vi "Keithley24xx_qMeasVil.vi"(5 "Vih, V":dbl, 6 "Vil, V":dbl, 7 "Voh, V":dbl, 8 "outVISA In":refnum<visa-resource-name>, 9 "outErr In":errorcluster, 10 "inVISA In":refnum<visa-resource-name>, 11 "inErr In":errorcluster) -> (0 "outVISA Out":refnum<visa-resource-name>, 1 "outErr Out":errorcluster, 2 "inVISA Out":refnum<visa-resource-name>, 3 "inErr Out":errorcluster, 4 "Vil meas, В":dbl format="%#.3g")   [LabVIEW 2014]
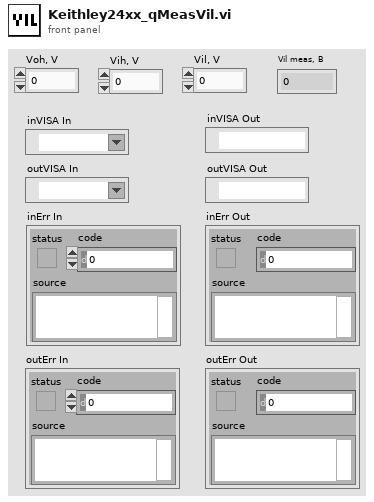
[diagram p1: front panel]
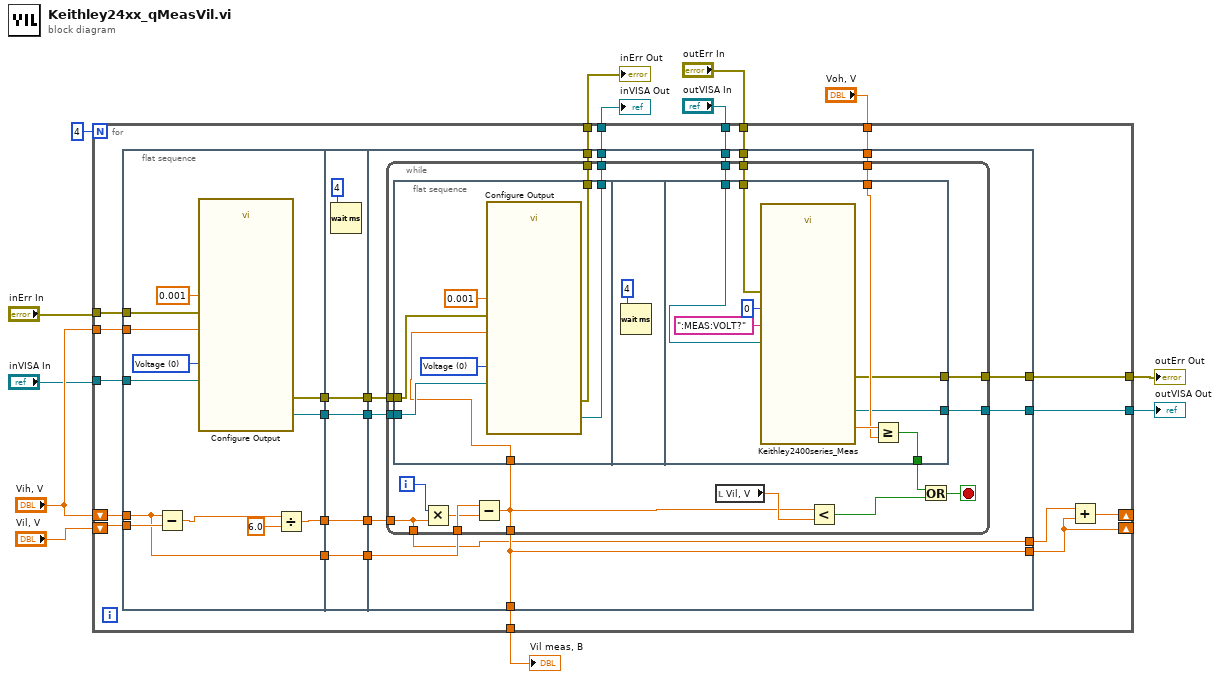
[diagram p0: block diagram]
diagram:
  n1 = for {
    N: 4 -> [_]
    shift-right: [w16] -> _
    shift-left: "Vih, V" -> [w31]
    shift-right: [w15] -> _
    shift-left: "Vil, V" -> [w32]
    tunnel: "Vih, V" -> [w29]
    tunnel: "Voh, V" -> [w28]
    tunnel: [w25] -> w9
    tunnel: "inErr In" -> [w24]
    tunnel: "inVISA In" -> [w23]
    tunnel: [w22] -> w6
    tunnel: [w21] -> w5
    tunnel: "outVISA In" -> [w20]
    tunnel: "outErr In" -> [w19]
    tunnel: [w18] -> w2
    tunnel: [w17] -> w1
    n2 = flat-sequence {
      tunnel: [w48] -> w37
      tunnel: [w47] -> w36
      tunnel: w31 -> [w40]
      tunnel: w32 -> [w45]
      tunnel: [w44] -> w30
      tunnel: w29 -> [w41]
      tunnel: [w40] -> w27
      tunnel: w24 -> [w39]
      tunnel: w23 -> [w38]
      tunnel: [w53] -> w35
      tunnel: w37 -> [w53]
      tunnel: [w52] -> w34
      tunnel: w36 -> [w52]
      tunnel: [w51] -> w33
      tunnel: w30 -> [w51]
      tunnel: w27 -> [w50]
      tunnel: [w50] -> w26
      tunnel: w35 -> [w67]
      tunnel: w34 -> [w66]
      tunnel: w33 -> [w65]
      tunnel: w28 -> [w64]
      tunnel: w26 -> [w63]
      tunnel: [w56] -> w25
      tunnel: [w62] -> w22
      tunnel: [w61] -> w21
      tunnel: w20 -> [w60]
      tunnel: w19 -> [w59]
      tunnel: [w58] -> w18
      tunnel: [w57] -> w17
      tunnel: [w56] -> w15
      tunnel: [w55] -> w14
      frame #0 {
        w49 = u16 0 items=["Voltage", "Current"] ("Source Mode  (0: Voltage)")
        n3 = Subtract(x=w40, y=w45) -> (x-y=w43:dbl)
        n4 = call "Configure Output.vi"("Source Mode  (0: Voltage)"=w49, "error in (no error)"=w39, "Compliance  Level (0.1)"=0.001, "Output Level (0)"=w41, "VISA resource name"=w38) -> ("error out"=w48:errorcluster, "VISA resource name out"=w47:refnum<visa-resource-name>)  [unwired: 5 in]
        n5 = Divide(x=w43, y=6.0) -> (x/y=w44:dbl)
      }
      frame #1 {
        n6 = Wait (ms)(milliseconds to wait=u32 4) -> ()  [unwired: 1 out]
      }
      frame #2 {
        n7 = while {
          tunnel: w67 -> [w82]
          tunnel: w66 -> [w81]
          tunnel: w65 -> [w68]
          tunnel: w64 -> [w79]
          tunnel: w63 -> [w78]
          tunnel: [w76] -> w56
          tunnel: [w74] -> w62
          tunnel: [w73] -> w61
          tunnel: w60 -> [w72]
          tunnel: w59 -> [w71]
          tunnel: [w70] -> w58
          tunnel: [w69] -> w57
          tunnel: [w68] -> w55
          i -> [w80]
          stop <- w85 stop-if-true
          n8 = flat-sequence {
            tunnel: w82 -> [w91]
            tunnel: w81 -> [w90]
            tunnel: w76 -> [w88]
            tunnel: [w87] -> w74
            tunnel: [w86] -> w73
            tunnel: [w100] -> w83
            tunnel: w79 -> [w98]
            tunnel: w72 -> [w97]
            tunnel: w71 -> [w96]
            tunnel: [w95] -> w70
            tunnel: [w94] -> w69
            frame #0 {
              w92 = u16 0 items=["Voltage", "Current"] ("Source Mode  (0: Voltage)")
              n9 = call "Configure Output.vi"("Source Mode  (0: Voltage)"=w92, "error in (no error)"=w91, "Compliance  Level (0.1)"=0.001, "Output Level (0)"=w88, "VISA resource name"=w90) -> ("error out"=w87:errorcluster, "VISA resource name out"=w86:refnum<visa-resource-name>)  [unwired: 5 in]
            }
            frame #1 {
              n10 = Wait (ms)(milliseconds to wait=u32 4) -> ()  [unwired: 1 out]
            }
            frame #2 {
              n11 = call "Keithley2400series_Meas.vi"("MEAS:<f>"=":MEAS:VOLT?", "error in (no error)"=w96, "MEAS mode, 0 Volt"=u16 0, "VISA resource name in"=w97) -> ("error out"=w95:errorcluster, "Замер"=w99:dbl, "VISA out"=w94:refnum<visa-resource-name>)  [unwired: 1 in, 1 out]
              n12 = Greater Or Equal?(x=w99, y=w98) -> (x >= y?=w100:bool)
            }
          }
          n13 = Multiply(x=w80, y=w68) -> (x*y=w75:dbl)
          n14 = Subtract(x=w78, y=w75) -> (x-y=w76:dbl)
          n15 = local read "Vil, V"() -> (w77:dbl)
          n16 = Less?(x=w76, y=w77) -> (x < y?=w84:bool)
          n17 = Or(x=w83, y=w84) -> (x .or. y?=w85:bool)
        }
      }
    }
    n18 = Add(x=w14, y=w15) -> (x+y=w16:dbl)
  }
  "Vil meas, В" <- w9
  "outVISA Out" <- w1
  "inVISA Out" <- w5
  "inErr Out" <- w6
  "outErr Out" <- w2
